vi "Role To Picture.vi"(11 "Role Data":string) -> (1 "Image Data":T1, 3 "Picture":picture)   [LabVIEW 2009, in "DSO1K.lvlib"]
doc: "Inputs the role data . Shows the new image and the image data information."
uses:
  <vilib>/picture/picture.llb/imagedata.ctl
  <instrlib>/DSO1K/DSO1K.lvlib
panel:
  in  "image data":T1
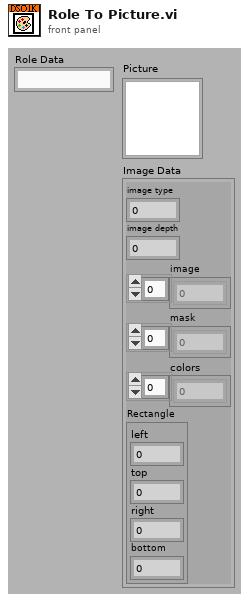
[diagram p1: front panel]
types:
  T1 = typedef "imagedata.ctl" = cluster{"image type":i32, "image depth":i32, "image":u8[], "mask":u8[], "colors":u32[], "Rectangle":cluster{"left":i16, "top":i16, "right":i16, "bottom":i16}}
  T2 = cluster{"left":i16, "top":i16, "right":i16, "bottom":i16}
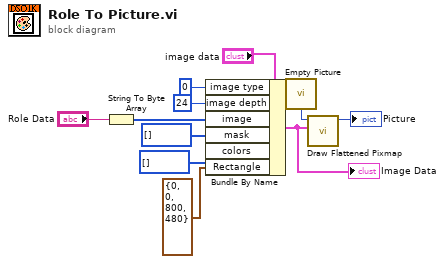
[diagram p0: block diagram]
diagram:
  n1 = String To Byte Array(string="Role Data") -> (unsigned byte array=w9:u8[])
  n2 = Bundle By Name(cluster="image data", "image type"=0, "image depth"=24, "image"=w9, "mask"=u8[] [], "colors"=u32[] [], "Rectangle"=T2 {"left"=0, "top"=0, "right"=800, "bottom"=480}) -> (w3:T1)
  "Image Data" <- w3
  n3 = call "Empty Picture"() -> ("empty picture"=w10:picture)
  n4 = call <vilib>:"Draw Flattened Pixmap.vi"("image data"=w3, "picture"=w10) -> ("new picture"=→"Picture":picture)  [unwired: 7 in]
